vi "status.get.vi"(8 "error in (no error)":errorcluster, 11 "midi-file-event.meta in":refnum<class "midi-file-event.meta.lvclass">) -> (0 "error out":errorcluster, 2 "MIDI Meta Events":T1, 3 "midi-file-event.meta out":refnum<class "midi-file-event.meta.lvclass">)   [LabVIEW 2020, in "midi-file-event.meta.lvclass"]
uses:
  midi-file-event.meta.lvclass
  midi-file/MIDI Meta Events.ctl
  midi-file-event.meta.lvclass/midi-file-event.meta.ctl
  midi-file/midi-file.lvclass
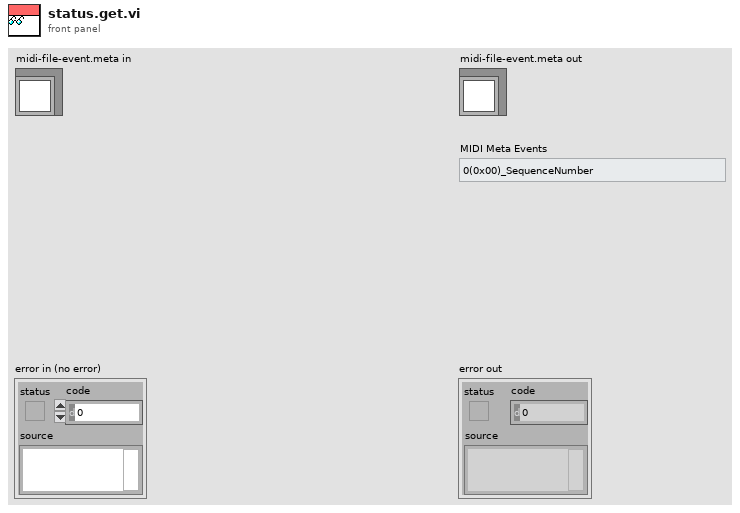
[diagram p1: front panel]
types:
  T1 = typedef "midi-file.lvclass/MIDI Meta Events.ctl" = enum8{"0(0x00)_SequenceNumber", "1(0x01)_TextEvent", "2(0x02)_CopyrightNotice", "3(0x03)_TrackOrSequenceName", "4(0x04)_InstrumentName", "5(0x05)_LyricText", "6(0x06)_MarkerText", "7(0x07)_CuePoint", "8(0x08)_UnassignedMetaEvent", "9(0x09)_UnassignedMetaEvent", "10(0x0A)_UnassignedMetaEvent", "11(0x0B)_UnassignedMetaEvent", "12(0x0C)_UnassignedMetaEvent", "13(0x0D)_UnassignedMetaEvent", "14(0x0E)_UnassignedMetaEvent", "15(0x0F)_UnassignedMetaEvent", "16(0x10)_UnassignedMetaEvent", "17(0x11)_UnassignedMetaEvent", "18(0x12)_UnassignedMetaEvent", "19(0x13)_UnassignedMetaEvent", "20(0x14)_UnassignedMetaEvent", "21(0x15)_UnassignedMetaEvent", "22(0x16)_UnassignedMetaEvent", "23(0x17)_UnassignedMetaEvent", "24(0x18)_UnassignedMetaEvent", "25(0x19)_UnassignedMetaEvent", "26(0x1A)_UnassignedMetaEvent", "27(0x1B)_UnassignedMetaEvent", "28(0x1C)_UnassignedMetaEvent", "29(0x1D)_UnassignedMetaEvent", "30(0x1E)_UnassignedMetaEvent", "31(0x1F)_UnassignedMetaEvent", "32(0x20)_MidiChannelPrefix", "33(0x21)_UnassignedMetaEvent", "34(0x22)_UnassignedMetaEvent", "35(0x23)_UnassignedMetaEvent", "36(0x24)_UnassignedMetaEvent", "37(0x25)_UnassignedMetaEvent", "38(0x26)_UnassignedMetaEvent", "39(0x27)_UnassignedMetaEvent", "40(0x28)_UnassignedMetaEvent", "41(0x29)_UnassignedMetaEvent", "42(0x2A)_UnassignedMetaEvent", "43(0x2B)_UnassignedMetaEvent", "44(0x2C)_UnassignedMetaEvent", "45(0x2D)_UnassignedMetaEvent", "46(0x2E)_UnassignedMetaEvent", "47(0x2F)_EndOfTrack", "48(0x30)_UnassignedMetaEvent", "49(0x31)_UnassignedMetaEvent", "50(0x32)_UnassignedMetaEvent", "51(0x33)_UnassignedMetaEvent", "52(0x34)_UnassignedMetaEvent", "53(0x35)_UnassignedMetaEvent", "54(0x36)_UnassignedMetaEvent", "55(0x37)_UnassignedMetaEvent", "56(0x38)_UnassignedMetaEvent", "57(0x39)_UnassignedMetaEvent", "58(0x3A)_UnassignedMetaEvent", "59(0x3B)_UnassignedMetaEvent", "60(0x3C)_UnassignedMetaEvent", "61(0x3D)_UnassignedMetaEvent", "62(0x3E)_UnassignedMetaEvent", "63(0x3F)_UnassignedMetaEvent", "64(0x40)_UnassignedMetaEvent", "65(0x41)_UnassignedMetaEvent", "66(0x42)_UnassignedMetaEvent", "67(0x43)_UnassignedMetaEvent", "68(0x44)_UnassignedMetaEvent", "69(0x45)_UnassignedMetaEvent", "70(0x46)_UnassignedMetaEvent", "71(0x47)_UnassignedMetaEvent", "72(0x48)_UnassignedMetaEvent", "73(0x49)_UnassignedMetaEvent", "74(0x4A)_UnassignedMetaEvent", "75(0x4B)_UnassignedMetaEvent", "76(0x4C)_UnassignedMetaEvent", "77(0x4D)_UnassignedMetaEvent", "78(0x4E)_UnassignedMetaEvent", "79(0x4F)_UnassignedMetaEvent", "80(0x50)_UnassignedMetaEvent", "81(0x51)_TempoSetting", "82(0x52)_UnassignedMetaEvent", "83(0x53)_UnassignedMetaEvent", "84(0x54)_SMPTEOffset", "85(0x55)_UnassignedMetaEvent", "86(0x56)_UnassignedMetaEvent", "87(0x57)_UnassignedMetaEvent", "88(0x58)_TimeSignature", "89(0x59)_KeySignature", "90(0x5A)_UnassignedMetaEvent", "91(0x5B)_UnassignedMetaEvent", "92(0x5C)_UnassignedMetaEvent", "93(0x5D)_UnassignedMetaEvent", "94(0x5E)_UnassignedMetaEvent", "95(0x5F)_UnassignedMetaEvent", "96(0x60)_UnassignedMetaEvent", "97(0x61)_UnassignedMetaEvent", "98(0x62)_UnassignedMetaEvent", "99(0x63)_UnassignedMetaEvent", "100(0x64)_UnassignedMetaEvent", "101(0x65)_UnassignedMetaEvent", "102(0x66)_UnassignedMetaEvent", "103(0x67)_UnassignedMetaEvent", "104(0x68)_UnassignedMetaEvent", "105(0x69)_UnassignedMetaEvent", "106(0x6A)_UnassignedMetaEvent", "107(0x6B)_UnassignedMetaEvent", "108(0x6C)_UnassignedMetaEvent", "109(0x6D)_UnassignedMetaEvent", "110(0x6E)_UnassignedMetaEvent", "111(0x6F)_UnassignedMetaEvent", "112(0x70)_UnassignedMetaEvent", "113(0x71)_UnassignedMetaEvent", "114(0x72)_UnassignedMetaEvent", "115(0x73)_UnassignedMetaEvent", "116(0x74)_UnassignedMetaEvent", "117(0x75)_UnassignedMetaEvent", "118(0x76)_UnassignedMetaEvent", "119(0x77)_UnassignedMetaEvent", "120(0x78)_UnassignedMetaEvent", "121(0x79)_UnassignedMetaEvent", "122(0x7A)_UnassignedMetaEvent", "123(0x7B)_UnassignedMetaEvent", "124(0x7C)_UnassignedMetaEvent", "125(0x7D)_UnassignedMetaEvent", "126(0x7E)_UnassignedMetaEvent", "127(0x7F)_SequencerSpecificMetaEvent"}
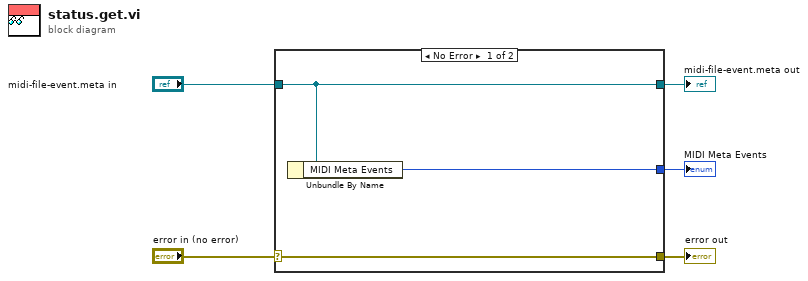
[diagram p0: block diagram]
diagram:
  n1 = case shown="No Error" "error in (no error)" {
    selector: "error in (no error)" -> [w8 w9]
    tunnel: [w8 w9] -> w4
    tunnel: [w7 w10] -> w2
    tunnel: "midi-file-event.meta in" -> [w7 w10]
    tunnel: [w6 _] -> w1
    frame No Error {
      n2 = Unbundle By Name(w7) -> ("MIDI Meta Events"=w6:T1)
    }
    frame Error {
    }
  }
  "error out" <- w4
  "midi-file-event.meta out" <- w2
  "MIDI Meta Events" <- w1
